vi "from string.vi"(8 "error in":errorcluster, 9 "data":string, 10 "version":string, 11 "tag bus configurable plugin module configuration in":refnum<class "tag bus configurable plugin module configuration.lvclass">) -> (0 "error out":errorcluster, 3 "tag bus configurable plugin module configuration out":refnum<class "tag bus configurable plugin module configuration.lvclass">)   [LabVIEW 2013, in "tag bus configurable plugin module configuration.lvclass"]
doc: "Provides an interface for loading a module configuration from a file or other serialized data source. It is recommended that all children of this class store data in two sets--data required for its own initialization, and any data required for parent initialization--and that each implementation uses the <b>Call Parent Method</b> primitive to de-serialize parent information. As a result, it is expected that every module configuration class calls <b>component configuration.lvclass:From String.vi</b>."
uses:
  tag bus configurable plugin module configuration.lvclass
  <vilib>/NI/Tag Bus Module Framework/module configuration/TBM module configuration.lvclass
  tag bus configurable plugin module configuration.lvclass/tag bus configurable plugin module configuration.ctl
  <vilib>/NI/Tag Bus Module Framework/root configuration/wrap data.vi
  <vilib>/NI/Tag Bus Module Framework/root configuration/create GUID.vi
  <vilib>/NI/Tag Bus Module Framework/channel/TBM channel.lvclass
  <vilib>/NI/Tag Bus Module Framework/root configuration/TBM configuration.lvclass
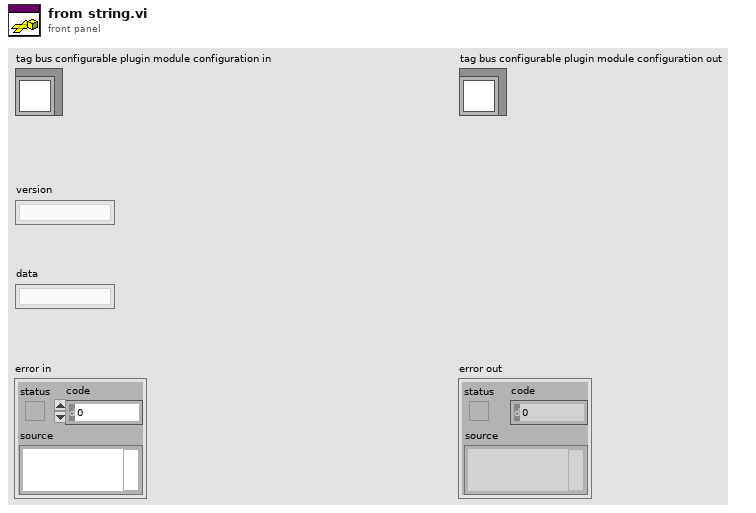
[diagram p1: front panel]
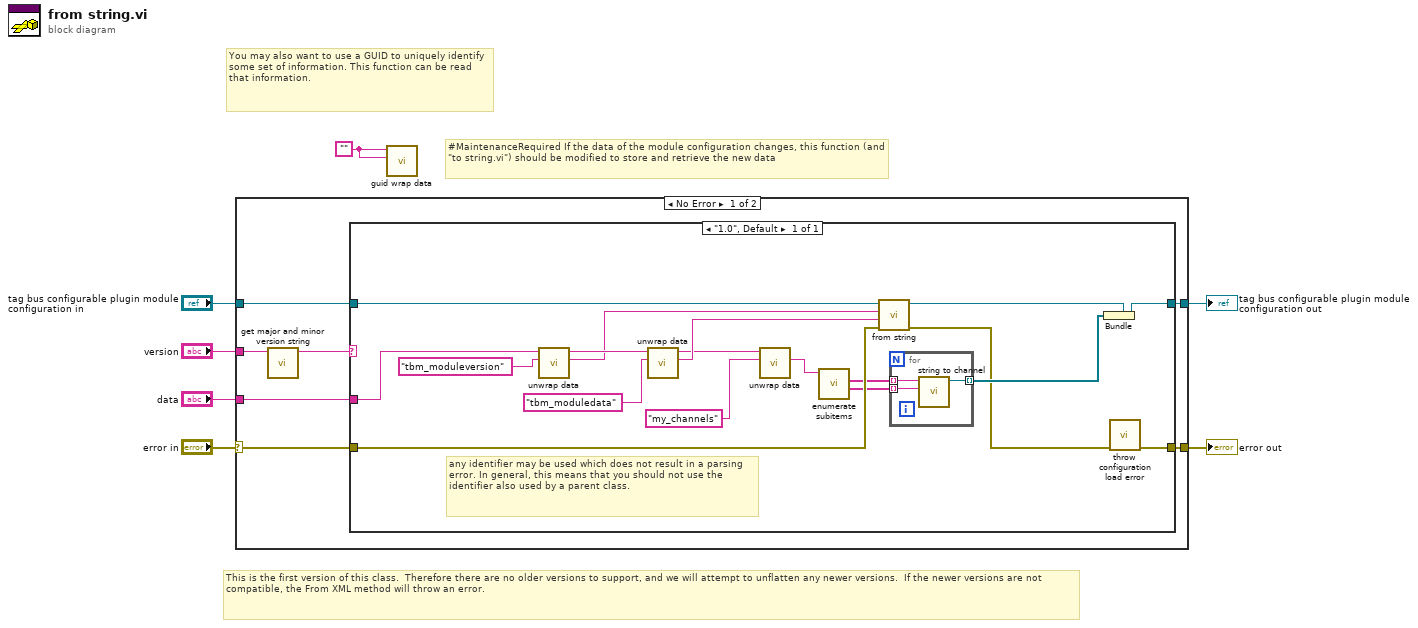
[diagram p0: block diagram]
diagram:
  w1 = ""
  # "You may also want to use a GUID to uniquely identify some set of information. This function can be read that information."
  # "#MaintenanceRequired If the data of the module configuration changes, this function (and \"to string.vi\") should be modified to store and retrieve the new data"
  # "This is the first version of this class.  Therefore there are no older versions to support, and we will attempt to unflatten any newer versions.  If the newer versions are not compatible, the From XML method will throw an error."
  n1 = case shown="No Error" "error in" {
    selector: "error in" -> [w8 w37]
    tunnel: "data" -> [w14 _]
    tunnel: "tag bus configurable plugin module configuration in" -> [w13 w36]
    tunnel: [w12 w36] -> w6
    tunnel: [w11 w37] -> w5
    tunnel: "version" -> [w10 _]
    frame No Error {
      n2 = call <vilib>:"get major and minor version string.vi"("full version"=w10) -> ("major.minor version"=w9:string)  [unwired: 10 in]
      n3 = case shown="\"1.0\", Default" w9 {
        tunnel: w14 -> [w28]
        tunnel: w8 -> [w27]
        tunnel: w13 -> [w32]
        tunnel: [w22] -> w12
        tunnel: [w30] -> w11
        frame "1.0", Default {
          # "any identifier may be used which does not result in a parsing error. In general, this means that you should not use the identifier also used by a parent class."
          n4 = call <vilib>:"unwrap data.vi"("identifier"="tbm_moduleversion" ("additional identifier"), "data to unwrap"=w28) -> ("unwrapped data"=w23:string, "remaining string"=w29:string)  [unwired: 8 in]
          n5 = call <vilib>:"unwrap data.vi"("identifier"="tbm_moduledata" ("additional identifier"), "data to unwrap"=w29) -> ("unwrapped data"=w25:string, "remaining string"=w21:string)  [unwired: 8 in]
          n6 = call <vilib>:"unwrap data.vi"("identifier"="my_channels" ("additional identifier"), "data to unwrap"=w21) -> ("unwrapped data"=w19:string)  [unwired: 8 in, 1 out]
          n7 = call <vilib>:"enumerate subitems.vi"("data to enumerate"=w19) -> ("associated data"=w17:string[], "discovered subitems"=w18:string[])  [unwired: 8 in, 1 out]
          n8 = call-parent "from string.vi"("error in"=w27, "data"=w25, "version"=w23, "module configuration in"=w32) -> ("error out"=w15:errorcluster, "module configuration out"=w31:refnum<class "tag bus configurable plugin module configuration.lvclass">)  [unwired: 6 in]
          n9 = for {
            tunnel: w18 -> [w35] mode=indexing
            tunnel: w17 -> [w34] mode=indexing
            tunnel: [w33] -> w16 mode=indexing
            n10 = call <vilib>:"string to channel.vi"("channel data"=w34, "identifier"=w35) -> ("channel in"=w33:refnum<class "TBM channel.lvclass">)  [unwired: 9 in]
          }
          n11 = Bundle(cluster=w31, w16) -> (w22:refnum<class "tag bus configurable plugin module configuration.lvclass">)
          n12 = call <vilib>:"throw configuration load error.vi"("error in"=w15) -> ("error out"=w30:errorcluster)  [unwired: 10 in]
        }
      }
    }
    frame Error {
    }
  }
  "error out" <- w5
  "tag bus configurable plugin module configuration out" <- w6
  n13 = call <vilib>:"guid wrap data.vi"("identifier"=w1, "data to wrap"=w1) -> ()  [unwired: 8 in, 2 out]
